vi "updateTupla.vi"(8 "error in":errorcluster, 9 "ItemNames":string[][](array[string]), 10 "RawIndexToModify":i32[](array[numeric]), 11 "tableName":string) -> (0 "error out":errorcluster)   [LabVIEW 2014]
uses:
  <vilib>/addons/database/Connection.llb/DB Tools Open Connec (String).vi
  <vilib>/addons/database/NI_Database_API.lvlib
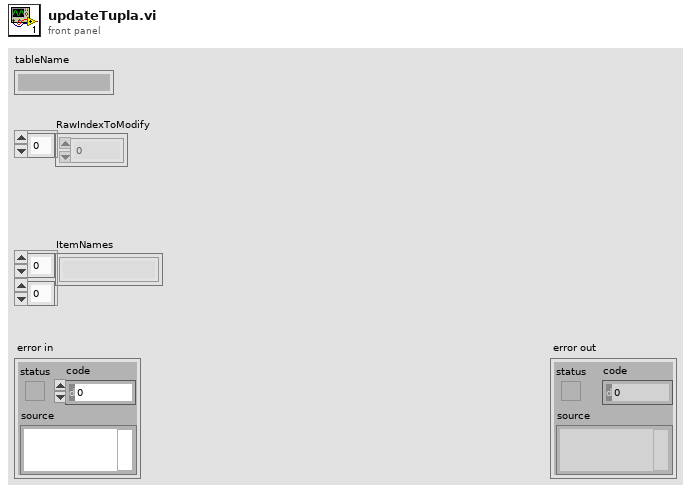
[diagram p1: front panel]
types:
  T1 = typedef "NI_Database_API.lvlib/Conn ObjectReference.ctl" = refnum<k1>
  T2 = typedef "NI_Database_API.lvlib/DB Tools DataTypes.ctl" = enum16{"String", "Long (I32)", "Single (SGL)", "Double (DBL)", "Date/Time", "Binary"}
  T3 = cluster{"name":string, "database data type":T2, "defined size":i32}[]
  T4 = cluster{cluster{string, string, string, string, string}, string[]}
  T5 = cluster{cluster{string, string, string}, string[]}
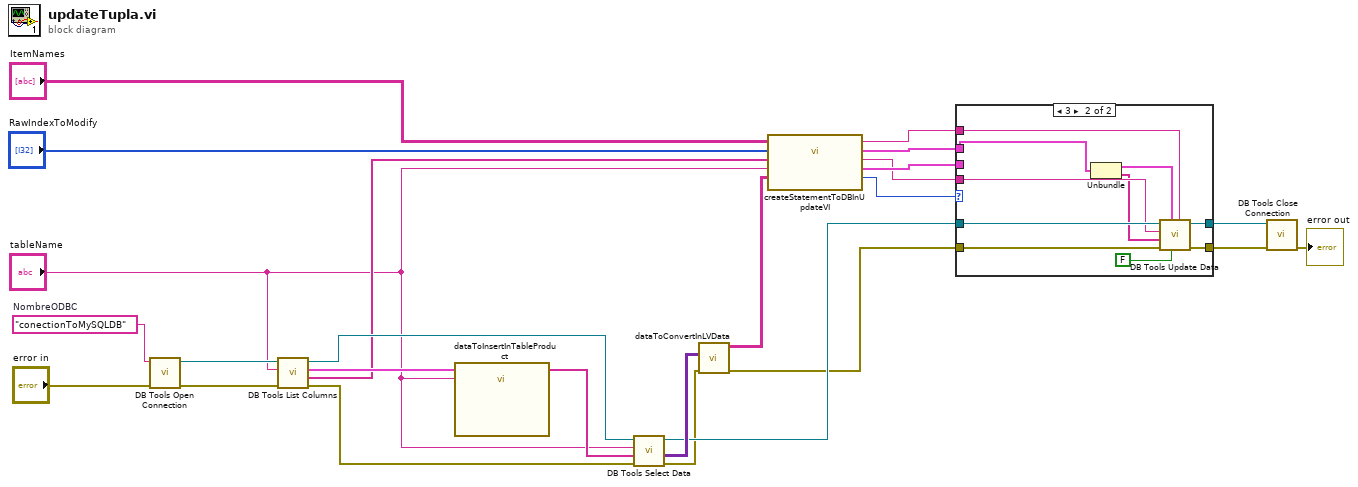
[diagram p0: block diagram]
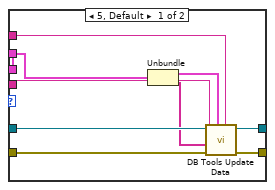
[diagram p2: hidden frame]
diagram:
  w19 = "conectionToMySQLDB"  # NombreODBC
  n1 = call-poly <vilib>:"DB Tools Open Connection.vi"("error in (no error)"="error in", "connection information"=w19) -> ("error out"=w9:errorcluster, "connection reference"=w10:T1)  [unwired: 6 in]
  n2 = call <vilib>:"DB Tools List Columns.vi"("error in (no error)"=w9, "table"="tableName", "connection reference"=w10) -> ("error out"=w13:errorcluster, "columns"=w7:string[], "column information"=w11:T3, "connection reference out"=w12:T1)  [unwired: 1 in]
  n3 = call "dataToInsertInTableProduct.vi"("arrayNamesInTableIN"=w11, "tableIn"="tableName") -> ("arrayNamesInTableOUT"=w15:string[])  [unwired: 7 in, 6 out]
  n4 = call <vilib>:"DB Tools Select Data.vi"("error in (no error)"=w13, "columns"=w15, "table"="tableName", "connection reference"=w12) -> ("error out"=w5:errorcluster, "data"=w14:variant[][], "connection reference out"=w8:T1)  [unwired: 2 in]
  n5 = call "dataToConvertInLVData.vi"("error in"=w5, "dataReadingIn"=w14) -> ("error out"=w4:errorcluster, "dataReadingOut"=w3:string[][])  [unwired: 8 in]
  n6 = call "createStatementToDBInUpdateVI.vi"("DataReadingInTableBeforeToUpdate"=w3, "Nombre Tabla"="tableName", "ColumnName"=w7, "RawIndexToModify"="RawIndexToModify", "ItemNames"="ItemNames") -> ("DataToModify5"=w23:T4, "TableNameToModify"=w22:string, "DataToModify3"=w24:T5, "statementSQL"=w25:string, "NumberOfFields"=w21:i32)  [unwired: 2 in]
  n7 = case shown="3" w21 {
    tunnel: w8 -> [w31 w44]
    tunnel: w4 -> [w32 w43]
    tunnel: [w33 w42] -> w17
    tunnel: [w34 w41] -> w16
    tunnel: w22 -> [w30 w40]
    tunnel: w25 -> [w29 w39]
    tunnel: w24 -> [_ w37]
    tunnel: w23 -> [w28 _]
    frame 5, Default {
      n8 = Unbundle(w28) -> (w27:cluster{string, string, string, string, string}, w26:string[])
      n9 = call <vilib>:"DB Tools Update Data.vi"("condition"=w29, "data"=w27, "error in (no error)"=w32, "columns"=w26, "table"=w30, "connection reference"=w31) -> ("error out"=w34:errorcluster, "connection reference out"=w33:T1)  [unwired: 4 in]
    }
    frame 3 {
      n10 = Unbundle(w37) -> (w36:cluster{string, string, string}, w35:string[])
      n11 = call <vilib>:"DB Tools Update Data.vi"("condition"=w39, "flatten cluster? (F)"=FALSE, "data"=w36, "error in (no error)"=w43, "columns"=w35, "table"=w40, "connection reference"=w44) -> ("error out"=w41:errorcluster, "connection reference out"=w42:T1)  [unwired: 3 in]
    }
  }
  n12 = call <vilib>:"DB Tools Close Connection.vi"("error in (no error)"=w16, "connection reference"=w17) -> ("error out"=→"error out":errorcluster)  [unwired: 5 in]
